vi "Send Response.vi"(0 "reference in":refnum<class "UE_slave.lvclass">, 1 "response":string, 2 "data":variant, 5 "error in (no error)":errorcluster) -> (14 "reference out":refnum<class "UE_slave.lvclass">, 19 "error out":errorcluster)   [LabVIEW 2019, in "CommandResponse communication.lvlib" / "UE_slave.lvclass"]
doc: "Sends response message to master. Should be called after recieving and processing command"
uses:
  UE_slave.lvclass
  Status + response + data cluster.ctl
  CommandResponse communication.lvlib
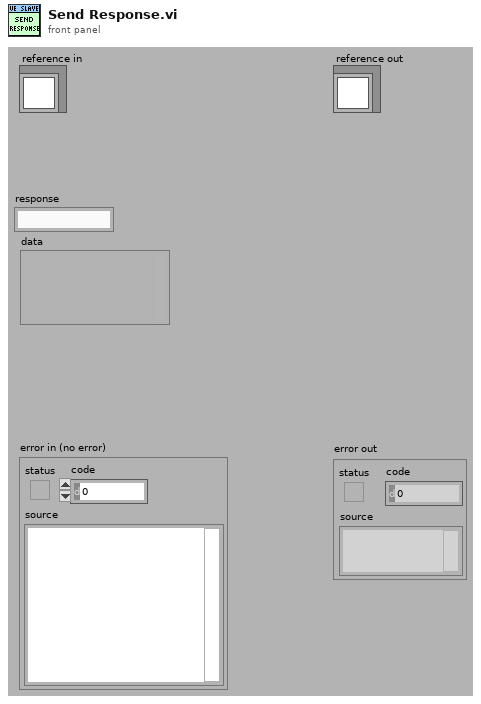
[diagram p1: front panel]
types:
  T1 = typedef "CommandResponse communication.lvlib/Status + response + data cluster.ctl" = cluster{"message":string, "response":string, "data":variant}
  T2 = typedef "CommandResponse communication.lvlib/UE_slave.lvclass/ObjectAttributes.ctl" = cluster{"response notifier":refnum<notifier>}
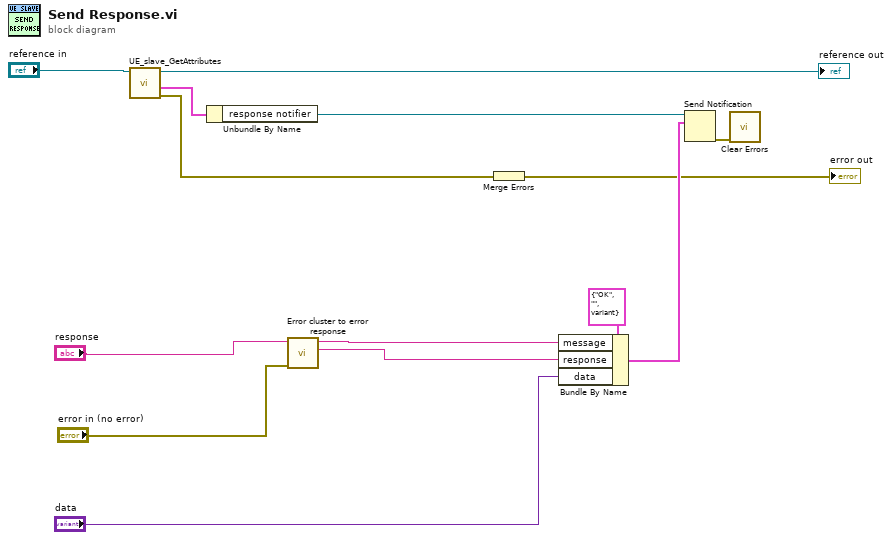
[diagram p0: block diagram]
diagram:
  n1 = call "UE_slave_GetAttributes.vi"("reference in"="reference in") -> ("error out"=w14:errorcluster, "attributes"=w9:T2, "reference out"=→"reference out":refnum<class "UE_slave.lvclass">)  [unwired: 7 in, 1 out]
  n2 = Unbundle By Name(w9) -> ("response notifier"=w8:refnum<notifier>)
  n3 = call "Error cluster to error response.vi"("error in (no error)"="error in (no error)", "response"="response") -> ("JSON String"=w1:string, "message"=w2:string)  [unwired: 7 in, 1 out]
  n4 = Merge Errors(w14) -> (→"error out":errorcluster)
  n5 = Bundle By Name(cluster=T1 {"message"="OK", "response"="", "data"=variant} ("notification"), "message"=w2, "response"=w1, "data"="data") -> (w6:T1)
  n6 = Send Notification(notification=w6, notifier=w8) -> (error out=w7:errorcluster)  [unwired: 1 in, 1 out]
  n7 = call <vilib>:"Clear Errors.vi"("error in (no error)"=w7) -> ()  [unwired: 5 in, 2 out]
